vi "create file headers.vi"(8 "error in":errorcluster, 11 "files":T1) -> (0 "error out":errorcluster, 3 "files  out":T1)   [LabVIEW 2017]
uses:
  typedefs/refnum cluster.ctl
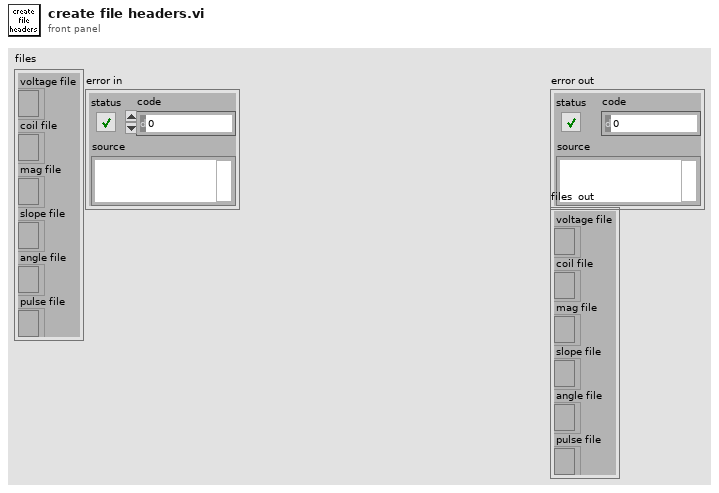
[diagram p1: front panel]
types:
  T1 = typedef "refnum cluster.ctl" = cluster{"voltage file":refnum<file>, "coil file":refnum<file>, "mag file":refnum<file>, "slope file":refnum<file>, "angle file":refnum<file>, "pulse file":refnum<file>}
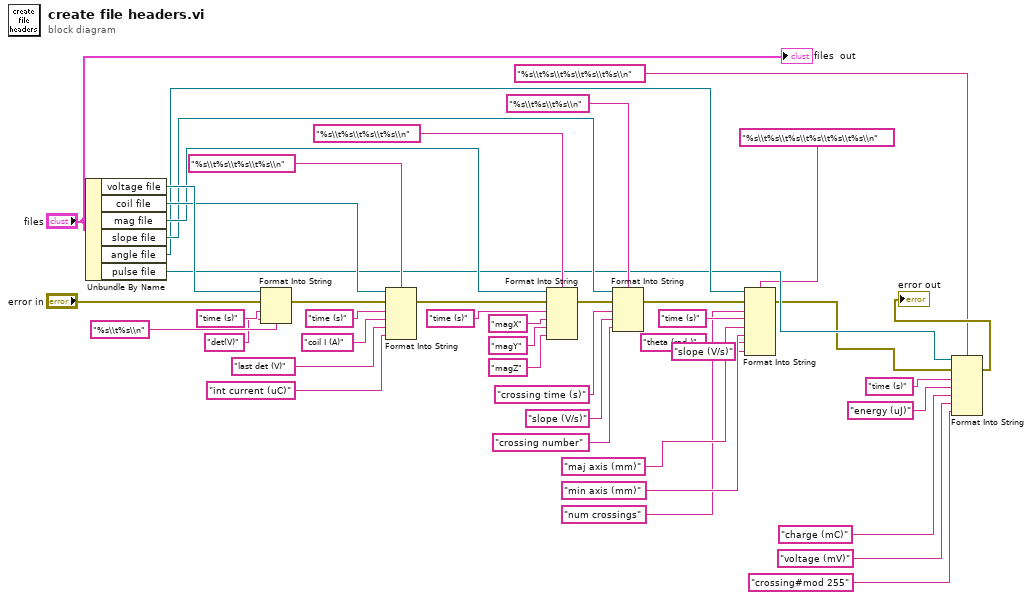
[diagram p0: block diagram]
diagram:
  n1 = Unbundle By Name("files") -> ("voltage file"=w43:refnum<file>, "coil file"=w36:refnum<file>, "mag file"=w25:refnum<file>, "slope file"=w20:refnum<file>, "angle file"=w19:refnum<file>, "pulse file"=w10:refnum<file>)
  n2 = Format Into String(format string="%s\\t%s\\n", initial string=w43, error in="error in", "time (s)" ("input 1"), "det(V)" ("input 2")) -> (error out=w33:errorcluster)  [unwired: 1 out]
  n3 = Format Into String(format string="%s\\t%s\\t%s\\t%s\\n", initial string=w36, error in=w33, "time (s)" ("input 1"), "coil I (A)" ("input 2"), "last det (V)" ("input 3"), "int current (uC)" ("input 4")) -> (error out=w26:errorcluster)  [unwired: 1 out]
  n4 = Format Into String(format string="%s\\t%s\\t%s\\t%s\\n", initial string=w25, error in=w26, "time (s)" ("input 1"), "magX" ("input 2"), "magY" ("input 3"), "magZ" ("input 4")) -> (error out=w17:errorcluster)  [unwired: 1 out]
  n5 = Format Into String(format string="%s\\t%s\\t%s\\n", initial string=w20, error in=w17, "crossing time (s)" ("input 1"), "slope (V/s)" ("input 2"), "crossing number" ("input 3")) -> (error out=w18:errorcluster)  [unwired: 1 out]
  n6 = Format Into String(format string="%s\\t%s\\t%s\\t%s\\t%s\\t%s\\n", initial string=w19, error in=w18, "num crossings" ("input 6"), "time (s)" ("input 1"), "maj axis (mm)" ("input 3"), "min axis (mm)" ("input 4"), "theta (rad )" ("input 2"), "slope (V/s)" ("input 6")) -> (error out=w9:errorcluster)  [unwired: 1 out]
  n7 = Format Into String(format string="%s\\t%s\\t%s\\t%s\\t%s\\n", initial string=w10, error in=w9, "time (s)" ("input 1"), "energy (uJ)" ("input 2"), "charge (mC)" ("input 3"), "voltage (mV)" ("input 4"), "crossing#mod 255" ("input 6")) -> (error out=→"error out":errorcluster)  [unwired: 1 out]
  "files  out" <- "files"
